vi "MoveGrip.vi"(8 "Close Grip":bool, 9 "Open Grip":bool, 10 "Close Limit Switch":bool, 11 "Open Limit Switch":bool) -> ()   [LabVIEW 2018]
uses:
  <vilib>/Rock Robotics/Network Tables/NT Write Boolean.vi
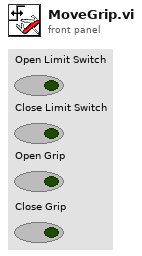
[diagram p1: front panel]
types:
  T1 = typedef "WPI_MotorControlDeviceRef.ctl" = cluster{"DeviceStatus":errorcluster, "Type":T2, "PWM":cluster{"PWM Channel":T3, "DeadBand":T4}, "CAN":cluster{"Device Number":u8, "SetOutput VI Ref":variant, "GetOutput VI Ref":variant, "Enable VI Ref":variant, "Disable VI Ref":variant, "Data":variant}, "Invert":bool, "DIO PWM":cluster{"PWM \"Enable\" Channel":T3, "DIOChannel":T5, "PWM Rate":dbl}}
  T2 = typedef "WPI_MotorControlType.ctl" = enum16{"PWM", "CAN", "DIO PWM"}
  T3 = typedef "FPGA_DIOPWMChannel.ctl" = enum8{"PWM 0", "PWM 1", "PWM 2", "PWM 3", "PWM 4", "PWM 5", "PWM 6", "PWM 7", "PWM 8", "PWM 9", "PWM MXP 0", "PWM MXP 1", "PWM MXP 2", "PWM MXP 3", "PWM MXP 4", "PWM MXP 5", "PWM MXP 6", "PWM MXP 7", "PWM MXP 8", "PWM MXP 9", "Invalid"}
  T4 = typedef "WPI_PWMDeadband.ctl" = cluster{"Name":string, "maxPositivePwm":i32, "minPositivePwm":i32, "centerPwm":i32, "maxNegativePwm":i32, "minNegativePwm":i32, "angularRange":u16}
  T5 = typedef "FPGA_DIOChannel.ctl" = enum8{"DIO 0", "DIO 1", "DIO 2", "DIO 3", "DIO 4", "DIO 5", "DIO 6", "DIO 7", "DIO 8", "DIO 9", "DIO MXP 0", "DIO MXP 1", "DIO MXP 2", "DIO MXP 3", "DIO MXP 4", "DIO MXP 5", "DIO MXP 6", "DIO MXP 7", "DIO MXP 8", "DIO MXP 9", "DIO MXP 10", "DIO MXP 11", "DIO MXP 12", "DIO MXP 13", "DIO MXP 14", "DIO MXP 15", "SPI Port CS1", "SPI Port CS2", "SPI Port CS3", "SPI Port MISO", "SPI Port MOSI", "Invalid"}
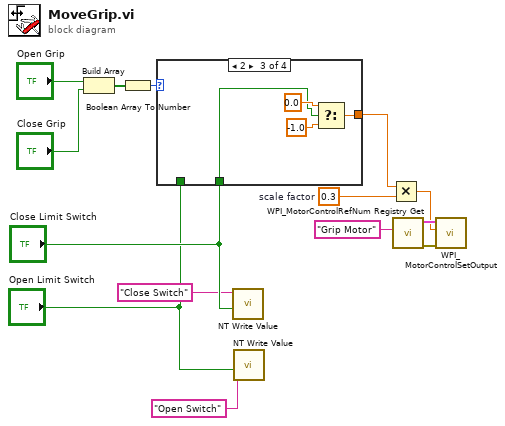
[diagram p0: block diagram]
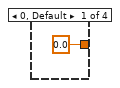
[diagram p2: hidden frame]
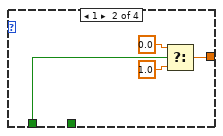
[diagram p3: hidden frame]
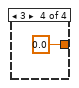
[diagram p4: hidden frame]
diagram:
  w5 = 0.3  # scale factor
  n1 = Build Array("Open Grip", "Close Grip") -> (w10:bool[])
  n2 = Boolean Array To Number(Boolean array=w10) -> (number=w9:u32)
  n3 = case shown="2" w9 {
    tunnel: [0.0 w17 w21 0.0] -> w8
    tunnel: "Close Limit Switch" -> [_ _ w20 _]
    tunnel: "Open Limit Switch" -> [_ w16 _ _]
    frame 0, Default {
    }
    frame 1 {
      n4 = Select(t=0.0, s=w16, f=1.0) -> (s? t:f=w17:dbl)
    }
    frame 2 {
      n5 = Select(t=0.0, s=w20, f=-1.0) -> (s? t:f=w21:dbl)
    }
    frame 3 {
    }
  }
  n6 = call-poly <vilib>:"NT Write Value.vi"("Boolean"="Close Limit Switch", "Name"="Close Switch") -> ()  [unwired: 9 in, 1 out]
  n7 = call-poly <vilib>:"NT Write Value.vi"("Boolean"="Open Limit Switch", "Name"="Open Switch") -> ()  [unwired: 9 in, 1 out]
  n8 = Multiply(x=w8, y=w5) -> (x*y=w6:dbl)
  n9 = call <vilib>:"WPI_MotorControlRefNum Registry Get.vi"("refnum name"="Grip Motor") -> ("error out"=w7:errorcluster, "MotorControlDevRef"=w13:T1)  [unwired: 9 in]
  n10 = call <vilib>:"WPI_MotorControlSetOutput.vi"("error in (no error)"=w7, "Output"=w6, "MotorControlDevRef"=w13) -> ()  [unwired: 6 in, 3 out]
